vi "Generate Profile.vi"(8 "error in (no error)":errorcluster, 11 "DCIR Parameters":T1 {"Pulse Mode" items=["Discharge"=1, "Charge"=2]; "Initial SoC (%)" min=0.0 max=100.0}) -> (0 "error out":errorcluster, 3 "DCIR Profile":waveform(dbl))   [LabVIEW 2023, in "DCIR_HPPC.lvclass"]
uses:
  DCIR_HPPC.lvclass
  HPPC Parameters.ctl
  HPPC Mode.ctl
  DCIR_HPPC.lvclass/DCIR_HPPC.ctl
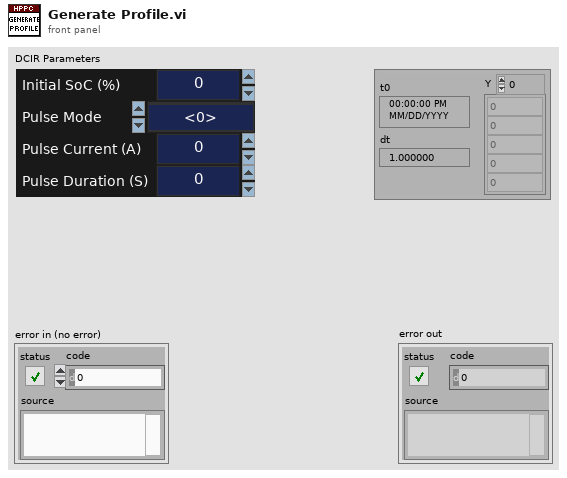
[diagram p1: front panel]
types:
  T1 = typedef "DCIR_HPPC.lvclass/HPPC Parameters.ctl" = cluster{"Initial SoC (%)":dbl, "Pulse Mode":T2, "Pulse Current (A)":dbl, "Pulse Duration (S)":dbl}
  T2 = typedef "DCIR_HPPC.lvclass/HPPC Mode.ctl" = u16
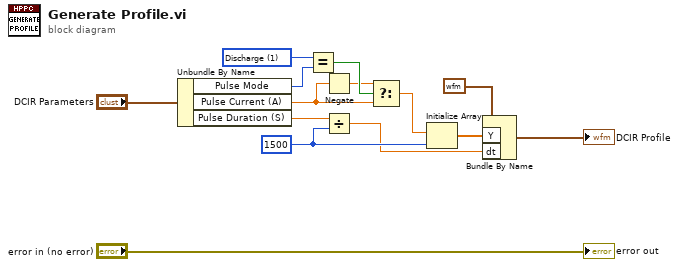
[diagram p0: block diagram]
diagram:
  w5 = 1500 ("dimension size")
  w12 = T2 1 items=["Discharge"=1, "Charge"=2] ("x")
  n1 = Unbundle By Name("DCIR Parameters") -> ("Pulse Mode"=w13:T2, "Pulse Current (A)"=w10:dbl, "Pulse Duration (S)"=w6:dbl)
  n2 = Equal?(x=w12, y=w13) -> (x = y?=w11:bool)
  n3 = Negate(x=w10) -> (-x=w9:dbl)
  n4 = Divide(x=w6, y=w5) -> (x/y=w3:dbl)
  n5 = Select(t=w9, s=w11, f=w10) -> (s? t:f=w7:dbl)
  n6 = Initialize Array(w7, w5) -> (w4:dbl[])
  n7 = Bundle By Name(cluster=waveform(dbl) {"t0"=timestamp(0 s since 1904-01-01), "dt"=1.0, "Y"=[]} ("waveform"), "Y"=w4, "dt"=w3) -> (→"DCIR Profile":waveform(dbl))
  "error out" <- "error in (no error)"
